vi "ChebyshevFitting.vi"(4 "Cernox_I":dbl, 6 "CernoxI measured with a lock-in?":bool=TRUE, 7 "Cernox T Fitting Control":T2, 8 "error in":errorcluster, 9 "2D Data Array In":dbl[][](array[numeric]), 10 "Title Name Array In":string[](array[string]), 11 "output cluster":T1={"Main Sweep"=0, "Steps Config:"={"total points:"=0, "Step Delay (s)"=0.0, "Ini Delay (s)"=0.0, "# of steps:"=0}, "Temperature Control (ITC 503):"={"GPIB ADR"=0, "Change Heater?"={"Heater?"=FALSE, "Heater"=0}, "Change Temp?"={"Change T?"=FALSE, "Set T (K)"=0.0}, "Cluster"={"Heat Auto?"=FALSE, "Manual Heat?"=FALSE, "Heater (%)"=0.0}, "Change PID?"={"Change PID?"=FALSE, "P"=0.0, "I"=0.0, "D"=0.0}, "Change Para?"=FALSE, "Sensor"=1}, "Temperature Control (LS 340):"={"GPIB ADR"=0, "From (K)"=0.0, "To (K)"=0.0, "Rate (K/min)"=0.0, "Delta T (0.08K)"=0.0, "Temp. Header"="", "T Display Control"={"Ch B"=FALSE, "Ch C"=FALSE, "Ch D"=FALSE}}, "Magnet Control (IPS 120-10)"={"Action"=0, "Standby (s)"=0.0, "Heater on (s)"=0.0, "Sweep Setup "=[], "GPIB ADR"=0, "Change Para?"=FALSE}, "Keithley 6221 :"=[], "Measuring Instruments : "=[], "Lock-In SR7265 :"=[], "Deascription of \nthis measurement"="", "Instruments Config:"=[], "LS372 Bridge : 2"=[{"GPIB"=0, "Excitation"=0, "Autorange?"=FALSE, "Range"=0, "Current"=0, "Voltage"=0, "DataHeader"="Rx;Ry"}], "Magnet Control (CS4) 2"={"Action"=1, "Standby (s)"=0.0, "Heater on (s)"=300.0, "Sweep Setup "=[], "GPIB ADR"=0, "Change Para?"=FALSE}} {"Magnet Control (CS4) 2"."GPIB ADR" items=["None"=0, "25"=25]; "Magnet Control (CS4) 2"."Sweep Setup"."Rate in Range (T/min)" min=0.001 max=0.5 step=0.001; "Magnet Control (CS4) 2"."Sweep Setup"."Hold(min)" min=0.0; "Magnet Control (CS4) 2"."Sweep Setup"."Set Point (T)" min=-9.0 max=9.0 step=0.001; "Magnet Control (CS4) 2"."Action" items=["Up", "Down", "Pause", "Zero"]; "LS372 Bridge : 2"."Voltage" items=["2.00 uV"=1, "6.32 uV"=2, "20.0 uV"=3, "63.2 uV"=4, "200 uV"=5, "632 uV"=6, "2.0 mV"=7, "6.32 mV"=8]; "LS372 Bridge : 2"."Current" items=["1.00 pA"=1, "3.16 pA"=2, "10.0 pA"=3, "31.6 pA"=4, "100 pA"=5, "316 pA"=6, "1.00 nA"=7, "3.16 nA"=8, "10 nA"=9, "31.6 nA"=10, "100 nA"=11, "316 nA"=12, "1.00 uA"=13, "3.16 uA"=14, "10.0 uA"=15, "31.6 uA"=16, "100 uA"=17, "316 uA"=18, "1.00 mA"=19, "3.16 mA"=20, "10.0 mA"=21, "31.6 mA"=22]; "LS372 Bridge : 2"."Range" items=["2.0 m"=1, "6.32 m"=2, "20.0 m"=3, "63.2 m"=4, "200 m"=5, "632 m"=6, "2.00"=7, "6.32"=8, "20.0"=9, "63.2"=10, "200"=11, "632"=12, "2.00 k"=13, "6.32 k"=14, "20.0 k"=15, "63.2 k"=16, "200 k"=17, "632 k"=18, "2.00 M"=19, "6.32 M"=20, "20.0 M"=21, "63.2 M"=22]; "LS372 Bridge : 2"."Excitation" items=["Voltage", "Current"]; "LS372 Bridge : 2"."GPIB" items=["None"=0, "9"=9]; "Main Sweep" items=["Time", "DC Current", "Delta Current", "Pulse Delta Current", "Sine Current", "Lock-in Vosc"]; "Temperature Control (ITC 503):"."Sensor" items=["T2", "T3"]; "Magnet Control (IPS 120-10)"."Action" items=["Hold", "To Set point", "To Zero", "Clamp"]; "Keithley 6221 :"."Sweep Mode" items=["Linear", "Log", "Exp", "Inverse", "Manual"]}) -> (0 "error out":errorcluster, 1 "2D Data ArrayOut":dbl[][](array[numeric]), 2 "Title Name Array Out":string[](array[string]), 3 "output cluster 2":T1={"Main Sweep"=0, "Steps Config:"={"total points:"=0, "Step Delay (s)"=0.0, "Ini Delay (s)"=0.0, "# of steps:"=0}, "Temperature Control (ITC 503):"={"GPIB ADR"=0, "Change Heater?"={"Heater?"=FALSE, "Heater"=0}, "Change Temp?"={"Change T?"=FALSE, "Set T (K)"=0.0}, "Cluster"={"Heat Auto?"=FALSE, "Manual Heat?"=FALSE, "Heater (%)"=0.0}, "Change PID?"={"Change PID?"=FALSE, "P"=0.0, "I"=0.0, "D"=0.0}, "Change Para?"=FALSE, "Sensor"=1}, "Temperature Control (LS 340):"={"GPIB ADR"=0, "From (K)"=0.0, "To (K)"=0.0, "Rate (K/min)"=0.0, "Delta T (0.08K)"=0.0, "Temp. Header"="", "T Display Control"={"Ch B"=FALSE, "Ch C"=FALSE, "Ch D"=FALSE}}, "Magnet Control (IPS 120-10)"={"Action"=0, "Standby (s)"=0.0, "Heater on (s)"=0.0, "Sweep Setup "=[], "GPIB ADR"=0, "Change Para?"=FALSE}, "Keithley 6221 :"=[], "Measuring Instruments : "=[], "Lock-In SR7265 :"=[], "Deascription of \nthis measurement"="", "Instruments Config:"=[], "LS372 Bridge : 2"=[{"GPIB"=0, "Excitation"=0, "Autorange?"=FALSE, "Range"=0, "Current"=0, "Voltage"=0, "DataHeader"="Rx;Ry"}], "Magnet Control (CS4) 2"={"Action"=1, "Standby (s)"=0.0, "Heater on (s)"=300.0, "Sweep Setup "=[], "GPIB ADR"=0, "Change Para?"=FALSE}} {"Magnet Control (CS4) 2"."GPIB ADR" items=["None"=0, "25"=25]; "Magnet Control (CS4) 2"."Sweep Setup"."Rate in Range (T/min)" min=0.001 max=0.5 step=0.001; "Magnet Control (CS4) 2"."Sweep Setup"."Hold(min)" min=0.0; "Magnet Control (CS4) 2"."Sweep Setup"."Set Point (T)" min=-9.0 max=9.0 step=0.001; "Magnet Control (CS4) 2"."Action" items=["Up", "Down", "Pause", "Zero"]; "LS372 Bridge : 2"."Voltage" items=["2.00 uV"=1, "6.32 uV"=2, "20.0 uV"=3, "63.2 uV"=4, "200 uV"=5, "632 uV"=6, "2.0 mV"=7, "6.32 mV"=8]; "LS372 Bridge : 2"."Current" items=["1.00 pA"=1, "3.16 pA"=2, "10.0 pA"=3, "31.6 pA"=4, "100 pA"=5, "316 pA"=6, "1.00 nA"=7, "3.16 nA"=8, "10 nA"=9, "31.6 nA"=10, "100 nA"=11, "316 nA"=12, "1.00 uA"=13, "3.16 uA"=14, "10.0 uA"=15, "31.6 uA"=16, "100 uA"=17, "316 uA"=18, "1.00 mA"=19, "3.16 mA"=20, "10.0 mA"=21, "31.6 mA"=22]; "LS372 Bridge : 2"."Range" items=["2.0 m"=1, "6.32 m"=2, "20.0 m"=3, "63.2 m"=4, "200 m"=5, "632 m"=6, "2.00"=7, "6.32"=8, "20.0"=9, "63.2"=10, "200"=11, "632"=12, "2.00 k"=13, "6.32 k"=14, "20.0 k"=15, "63.2 k"=16, "200 k"=17, "632 k"=18, "2.00 M"=19, "6.32 M"=20, "20.0 M"=21, "63.2 M"=22]; "LS372 Bridge : 2"."Excitation" items=["Voltage", "Current"]; "LS372 Bridge : 2"."GPIB" items=["None"=0, "9"=9]; "Main Sweep" items=["Time", "DC Current", "Delta Current", "Pulse Delta Current", "Sine Current", "Lock-in Vosc"]; "Temperature Control (ITC 503):"."Sensor" items=["T2", "T3"]; "Magnet Control (IPS 120-10)"."Action" items=["Hold", "To Set point", "To Zero", "Clamp"]; "Keithley 6221 :"."Sweep Mode" items=["Linear", "Log", "Exp", "Inverse", "Manual"]})   [LabVIEW 2012]
panel:
  out "Cernox T":dbl[](array[numeric])
  out "Cernox R":dbl[](array[numeric])
  out "Cernox I index":i32
  out "Cernox V index":i32
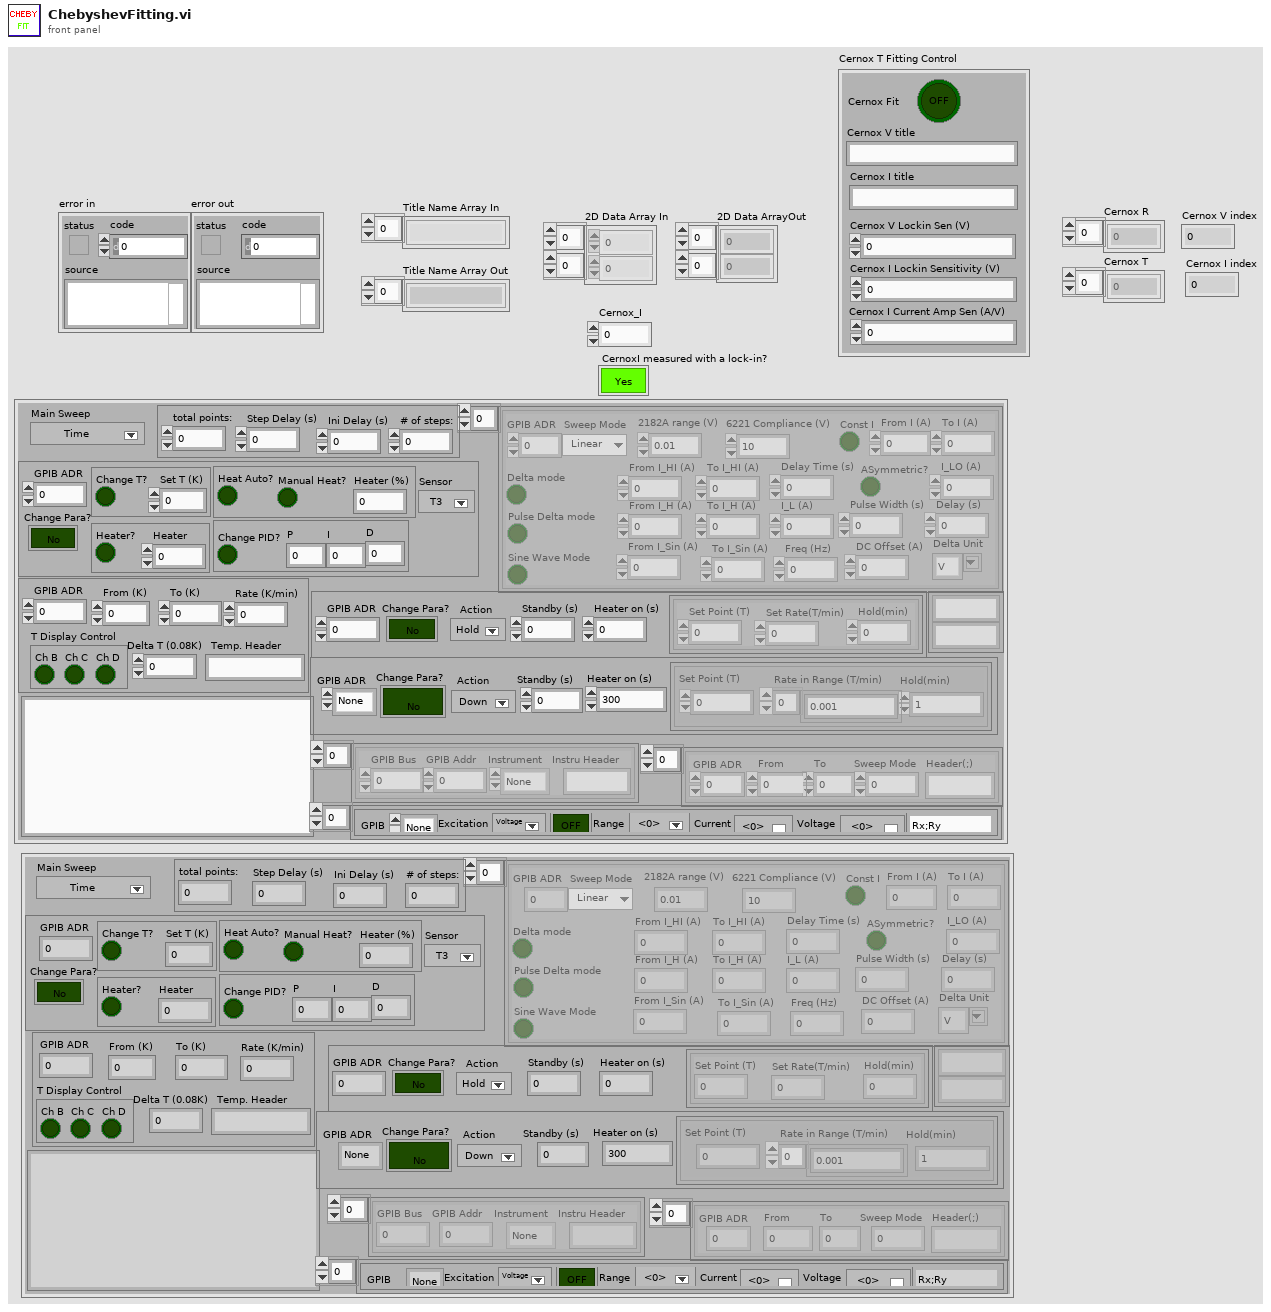
[diagram p1: front panel]
types:
  T1 = cluster{"Main Sweep":u8, "Steps Config:":cluster{"total points:":u32, "Step Delay (s)":dbl, "Ini Delay (s)":dbl, "# of steps:":u32}, "Temperature Control (ITC 503):":cluster{"GPIB ADR":u16, "Change Heater?":cluster{"Heater?":bool, "Heater":u8}, "Change Temp?":cluster{"Change T?":bool, "Set T (K)":dbl}, "Cluster":cluster{"Heat Auto?":bool, "Manual Heat?":bool, "Heater (%)":dbl}, "Change PID?":cluster{"Change PID?":bool, "P":dbl, "I":dbl, "D":dbl}, "Change Para?":bool, "Sensor":u16}, "Temperature Control (LS 340):":cluster{"GPIB ADR":u16, "From (K)":dbl, "To (K)":dbl, "Rate (K/min)":dbl, "Delta T (0.08K)":dbl, "Temp. Header":string, "T Display Control":cluster{"Ch B":bool, "Ch C":bool, "Ch D":bool}}, "Magnet Control (IPS 120-10)":cluster{"Action":u16, "Standby (s)":dbl, "Heater on (s)":dbl, "Sweep Setup ":cluster{"Set Point (T)":dbl, "Set Rate(T/min)":dbl, "Hold(min)":dbl}[], "GPIB ADR":u16, "Change Para?":bool}, "Keithley 6221 :":cluster{"Delta mode":bool, "Const I":bool, "Pulse Delta mode":bool, "Sine Wave Mode":bool, "From I_HI (A)":dbl, "From I (A)":dbl, "I_LO (A)":dbl, "From I_H (A)":dbl, "I_L (A)":dbl, "Freq (Hz)":dbl, "From I_Sin (A)":dbl, "DC Offset (A)":dbl, "Delay Time (s)":dbl, "Pulse Width (s)":dbl, "Delay (s)":dbl, "To I (A)":dbl, "ASymmetric?":bool, "To I_HI (A)":dbl, "To I_H (A)":dbl, "To I_Sin (A)":dbl, "GPIB ADR":u16, "Sweep Mode":u8, "Delta Unit":string, "2182A range (V)":dbl, "6221 Compliance (V)":dbl}[], "Measuring Instruments : ":cluster{"GPIB Bus":dbl, "GPIB Addr":dbl, "Instrument":enum16{"None", "HP34401DMM", "Lockin 7265", "HP3456/7A", "HP3478A", "HP3325FG", "Keithley2182A"}, "Instru Header":string}[], "Lock-In SR7265 :":cluster{"GPIB ADR":u16, "From":dbl, "To":dbl, "Header(;)":string, "Sweep Mode":u8}[], "Deascription of \nthis measurement":string, "Instruments Config:":string[][], "LS372 Bridge : 2":cluster{"GPIB":u16, "Excitation":u16, "Autorange?":bool, "Range":u16, "Current":u16, "Voltage":u16, "DataHeader":string}[], "Magnet Control (CS4) 2":cluster{"Action":u16, "Standby (s)":dbl, "Heater on (s)":dbl, "Sweep Setup ":cluster{"Set Point (T)":dbl, "Hold(min)":dbl, "Rate in Range (T/min)":dbl[]}[], "GPIB ADR":u16, "Change Para?":bool}}
  T2 = cluster{"Cernox V title":string, "Cernox I title":string, "Cernox V Lockin Sen (V)":dbl, "Cernox I Lockin Sensitivity (V)":dbl, "Cernox I Current Amp Sen (A/V)":dbl, "Cernox Fit":bool}
  T3 = cluster{"GPIB ADR":u16, "From":dbl, "To":dbl, "Header(;)":string, "Sweep Mode":u8}[]
  T4 = cluster{"GPIB Bus":dbl, "GPIB Addr":dbl, "Instrument":enum16{"None", "HP34401DMM", "Lockin 7265", "HP3456/7A", "HP3478A", "HP3325FG", "Keithley2182A"}, "Instru Header":string}[]
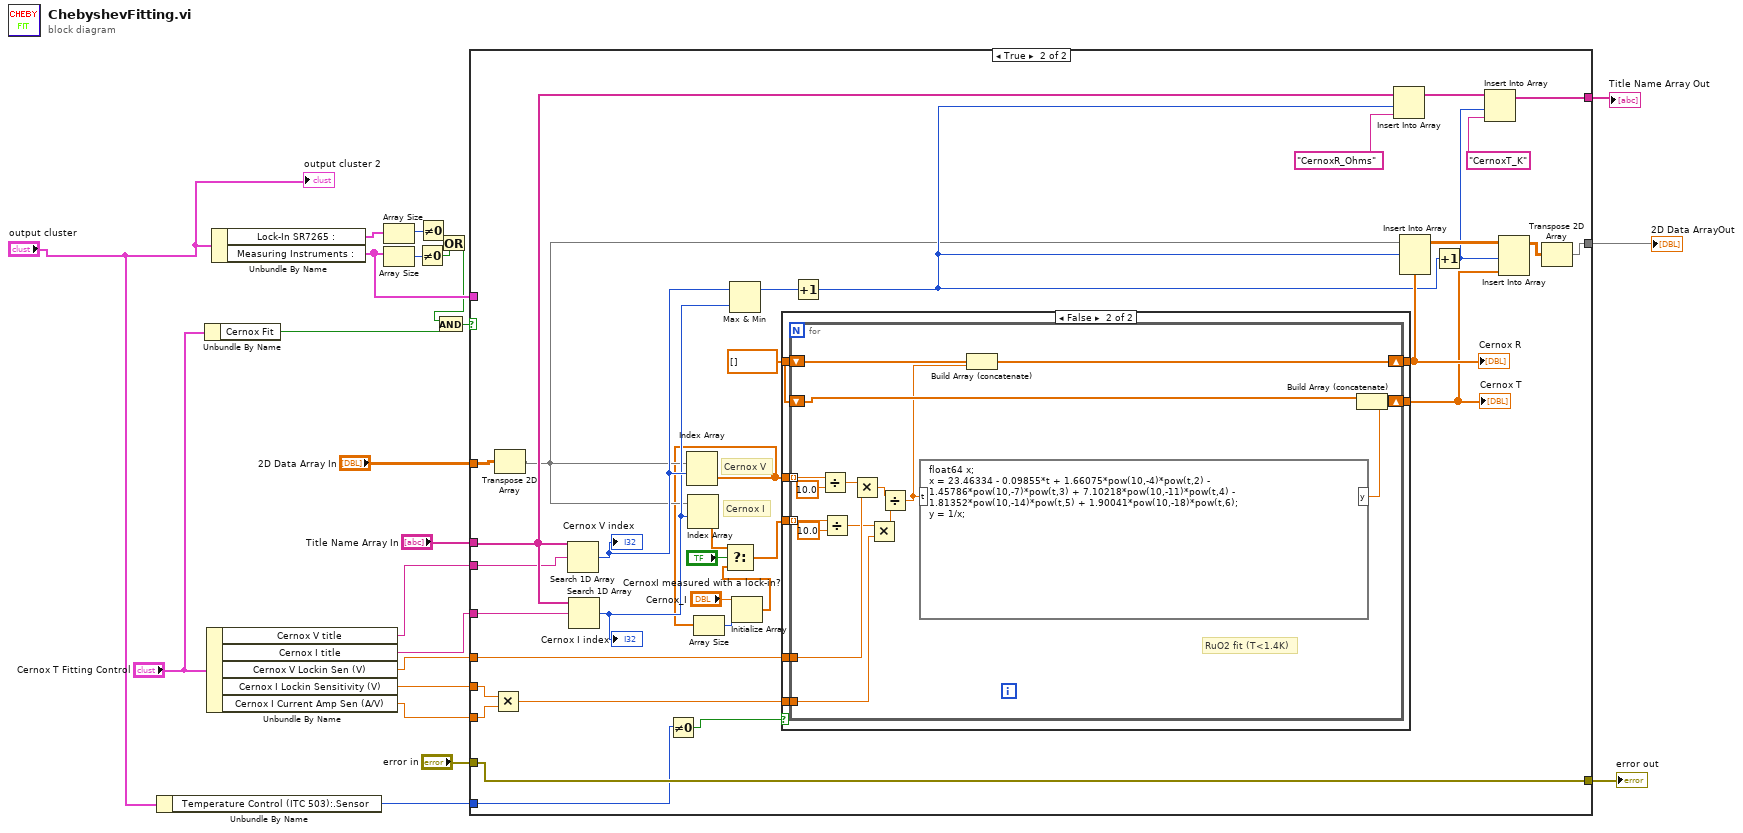
[diagram p0: block diagram]
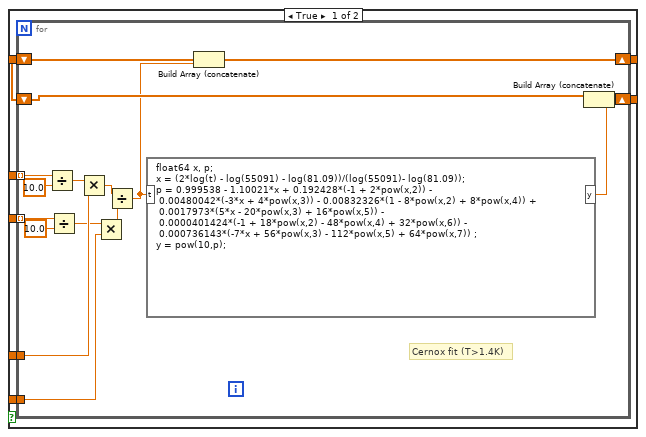
[diagram p3: hidden frame]
diagram:
  n1 = Unbundle By Name("output cluster") -> ("Temperature Control (ITC 503):.Sensor"=w2:u16)
  n2 = Unbundle By Name("Cernox T Fitting Control") -> ("Cernox Fit"=w10:bool)
  n3 = Unbundle By Name("Cernox T Fitting Control") -> ("Cernox V title"=w13:string, "Cernox I title"=w12:string, "Cernox V Lockin Sen (V)"=w16:dbl, "Cernox I Lockin Sensitivity (V)"=w15:dbl, "Cernox I Current Amp Sen (A/V)"=w14:dbl)
  n4 = Unbundle By Name("output cluster") -> ("Lock-In SR7265 :"=w7:T3, "Measuring Instruments :"=w22:T4)
  n5 = Array Size(array=w7) -> (size(s)=w6:i32)
  n6 = Array Size(array=w22) -> (size(s)=w23:i32)
  n7 = Not Equal To 0?(x=w23) -> (x != 0?=w4:bool)
  n8 = Not Equal To 0?(x=w6) -> (x != 0?=w5:bool)
  n9 = Or(x=w5, y=w4) -> (x .or. y?=w3:bool)
  n10 = And(x=w3, y=w10) -> (x .and. y?=w9:bool)
  n11 = case shown="True" w9 {
    tunnel: w22 -> [_ _]
    tunnel: "Title Name Array In" -> [w26 w49]
    tunnel: w16 -> [_ w60]
    tunnel: w15 -> [_ w59]
    tunnel: w14 -> [_ w58]
    tunnel: [w24 w36] -> w20
    tunnel: [w26 w43] -> w19
    tunnel: "error in" -> [w25 w42]
    tunnel: [w25 w42] -> w17
    tunnel: w13 -> [_ w41]
    tunnel: w12 -> [_ w40]
    tunnel: "2D Data Array In" -> [w24 w38]
    tunnel: w2 -> [_ w34]
    frame False {
    }
    frame True {
      # "Cernox I"
      # "Cernox V"
      n12 = Multiply(x=w59, y=w58) -> (x*y=w57:dbl)
      n13 = Transpose 2D Array(2D array=w38) -> (transposed array=w39:dbl[][])
      n14 = Search 1D Array(1D array=w49, element=w41) -> (index of element=w54:i32)  [unwired: 1 in]
      "Cernox V index" <- w54
      n15 = Search 1D Array(1D array=w49, element=w40) -> (index of element=w53:i32)  [unwired: 1 in]
      "Cernox I index" <- w53
      n16 = Not Equal To 0?(x=w34) -> (x != 0?=w35:bool)
      n17 = Index Array(array=w39, index (row)=w54) -> (element=w28:dbl[])  [unwired: 1 in]
      n18 = Index Array(array=w39, index (row)=w53) -> (element=w33:dbl[])  [unwired: 1 in]
      n19 = Array Size(array=w28) -> (size(s)=w30:i32)
      n20 = Max & Min(x=w54, y=w53) -> (max(x,y)=w52:i32)  [unwired: 1 out]
      n21 = Initialize Array("Cernox_I", w30) -> (w29:dbl[])
      n22 = Select(t=w33, s="CernoxI measured with a lock-in?", f=w29) -> (s? t:f=w32:dbl[])
      n23 = case shown="False" w35 {
        tunnel: w28 -> [w67 w90]
        tunnel: w32 -> [w66 w89]
        tunnel: w60 -> [w65 w88]
        tunnel: w57 -> [w64 w87]
        tunnel: dbl[] [] ("subarray") -> [w63 w86]
        tunnel: [w62 w85] -> w55
        tunnel: [w61 w84] -> w50
        frame True {
          n24 = for {
            tunnel: w67 -> [w81] mode=indexing
            tunnel: w66 -> [w77] mode=indexing
            shift-right: [w82] -> w62
            shift-left: w63 -> [w83]
            tunnel: w65 -> [w78]
            tunnel: w64 -> [w74]
            shift-right: [w70] -> w61
            shift-left: w63 -> [w71]
            # "Cernox fit (T>1.4K)"
            n25 = Divide(x=w81, y=10.0) -> (x/y=w79:dbl)
            n26 = Divide(x=w77, y=10.0) -> (x/y=w75:dbl)
            n27 = Multiply(x=w79, y=w78) -> (x*y=w73:dbl)
            n28 = Multiply(x=w75, y=w74) -> (x*y=w72:dbl)
            n29 = Divide(x=w73, y=w72) -> (x/y=w69:dbl)
            n30 = formula code="float64 x, p;\nx = (2*log(t) - log(55091) - log(81.09))/(log(55091)- log(81.09));\np = 0.999538 - 1.10021*x + 0.192428*(-1 + 2*pow(x,2)) - \n 0.00480042*(-3*x + 4*pow(x,3)) - 0.00832326*(1 - 8*pow(x,2) + 8*pow(x,4)) + \n 0.0017973*(5*x - 20*pow(x,3) + 16*pow(x,5)) - \n 0.0000401424*(-1 + 18*pow(x,2) - 48*pow(x,4) + 32*pow(x,6)) - \n 0.000736143*(-7*x + 56*pow(x,3) - 112*pow(x,5) + 64*pow(x,7)) ;\ny = pow(10,p);"("t"=w69) -> ("y"=w68:dbl)
            n31 = Build Array (concatenate)(w83, w69) -> (w82:dbl[])
            n32 = Build Array (concatenate)(w71, w68) -> (w70:dbl[])
          }
        }
        frame False {
          n33 = for {
            tunnel: w90 -> [w104] mode=indexing
            tunnel: w89 -> [w100] mode=indexing
            shift-right: [w105] -> w85
            shift-left: w86 -> [w106]
            tunnel: w88 -> [w101]
            tunnel: w87 -> [w97]
            shift-right: [w93] -> w84
            shift-left: w86 -> [w94]
            # "RuO2 fit (T<1.4K)"
            n34 = Divide(x=w104, y=10.0) -> (x/y=w102:dbl)
            n35 = Divide(x=w100, y=10.0) -> (x/y=w98:dbl)
            n36 = Multiply(x=w102, y=w101) -> (x*y=w96:dbl)
            n37 = Multiply(x=w98, y=w97) -> (x*y=w95:dbl)
            n38 = Divide(x=w96, y=w95) -> (x/y=w92:dbl)
            n39 = formula code="float64 x;\nx = 23.46334 - 0.09855*t + 1.66075*pow(10,-4)*pow(t,2) - \n1.45786*pow(10,-7)*pow(t,3) + 7.10218*pow(10,-11)*pow(t,4) - \n1.81352*pow(10,-14)*pow(t,5) + 1.90041*pow(10,-18)*pow(t,6);\ny = 1/x;"("t"=w92) -> ("y"=w91:dbl)
            n40 = Build Array (concatenate)(w106, w92) -> (w105:dbl[])
            n41 = Build Array (concatenate)(w94, w91) -> (w93:dbl[])
          }
        }
      }
      "Cernox R" <- w55
      "Cernox T" <- w50
      n42 = Increment(x=w52) -> (x+1=w48:i32)
      n43 = Insert Into Array(array=w49, index=w48, new element="CernoxR_Ohms" ("new element/subarray")) -> (w47:string[])
      n44 = Insert Into Array(array=w39, index (row)=w48, new element=w55) -> (w51:dbl[][])  [unwired: 1 in]
      n45 = Increment(x=w48) -> (x+1=w44:i32)
      n46 = Insert Into Array(array=w47, index=w44, new element="CernoxT_K" ("new element/subarray")) -> (w43:string[])
      n47 = Insert Into Array(array=w51, index (row)=w44, new element=w50) -> (w37:dbl[][])  [unwired: 1 in]
      n48 = Transpose 2D Array(2D array=w37) -> (transposed array=w36:dbl[][])
    }
  }
  "error out" <- w17
  "2D Data ArrayOut" <- w20
  "Title Name Array Out" <- w19
  "output cluster 2" <- "output cluster"
